vi "StateController.vi"(1 "Selected State (In)":string) -> (0 "Selected State (Out)":string)   [LabVIEW 2019]
uses:
  outputs.vi
panel:
  out "State Index":i32
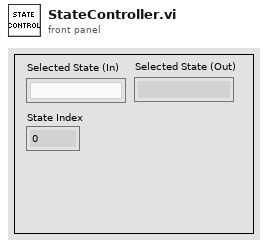
[diagram p1: front panel]
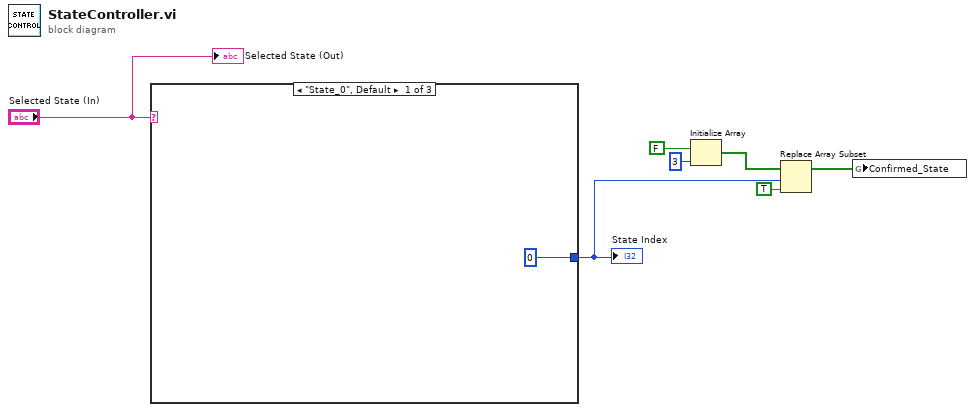
[diagram p0: block diagram]
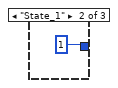
[diagram p2: hidden frame]
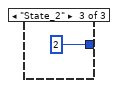
[diagram p3: hidden frame]
diagram:
  n1 = case shown="\"State_0\", Default" "Selected State (In)" {
    tunnel: [0 ("Index") 1 ("Index") 2 ("Index")] -> w3
    frame "State_0", Default {
    }
    frame "State_1" {
    }
    frame "State_2" {
    }
  }
  "State Index" <- w3
  n2 = Initialize Array(FALSE, 3 ("dimension size")) -> (w4:bool[])
  n3 = Replace Array Subset(array=w4, new element=TRUE ("new element/subarray"), index=w3) -> (w1:bool[])
  n4 = global write "outputs.vi" "Confirmed_State"(w1) -> ()
  "Selected State (Out)" <- "Selected State (In)"
